vi "To Variant.vi"(8 "Error In":errorcluster, 11 "TD Error Cluster":refnum<class "Error Cluster.lvclass">) -> (0 "Error Out":errorcluster, 2 "Variant":variant)   [LabVIEW 2020, in "NI_VIAnCFGDataStructure.lvlib" / "Error Cluster.lvclass"]
doc: "Dynamic dispatch interface for conversion of Tree Data classes to variant LV data."
uses:
  <vilib>/addons/analyzer/VIAnCFGDataStructure/Data Types/Error Cluster/Error Cluster.lvclass
  <vilib>/addons/analyzer/VIAnCFGDataStructure/Data Types/Error Cluster/Error Cluster.lvclass/Error Cluster.ctl
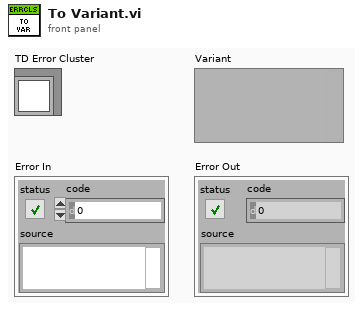
[diagram p1: front panel]
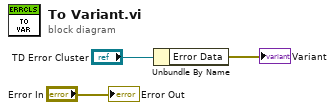
[diagram p0: block diagram]
diagram:
  n1 = Unbundle By Name("TD Error Cluster") -> ("Error Data"=→"Variant":errorcluster)
  "Error Out" <- "Error In"
